vi "LabVIEW2018_RS232_loopback_test.vi"() -> ()   [LabVIEW 2018]
uses:
  <vilib>/Instr/_visa.llb/VISA Configure Serial Port (Instr).vi
panel:
  in  "Delay Time (s)":dbl=0.5 format="%#_13g"
  in  "Send":bool
  in  "Flow control":u16(ring) items=["None", "XON/XOFF", "RTS/CTS", "XON/XOFF & RTS/CTS", "DTR/DSR", "XON/XOFF & DTR/DSR"]
  in  "Stop bits":u16(ring)=10 items=["1.0"=10, "1.5"=15, "2.0"=20]
  in  "Parity":enum16{"None", "Odd", "Even", "Mark", "Space"}(ring)
  in  "Data bits":u16=8
  in  "Baud rate":u32=9600
  in  "Sent Message":string="meas1?"
  in  "VISA resource name":refnum<visa-resource-name>="COM3"
  out "Read Response":string
  in  "stop":bool
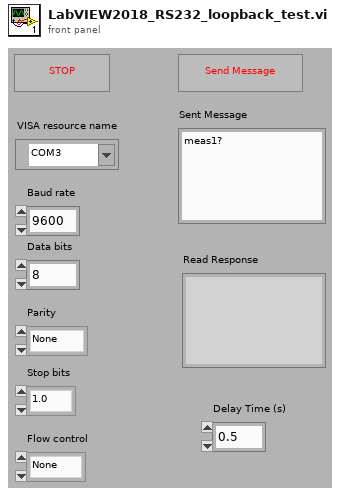
[diagram p1: front panel]
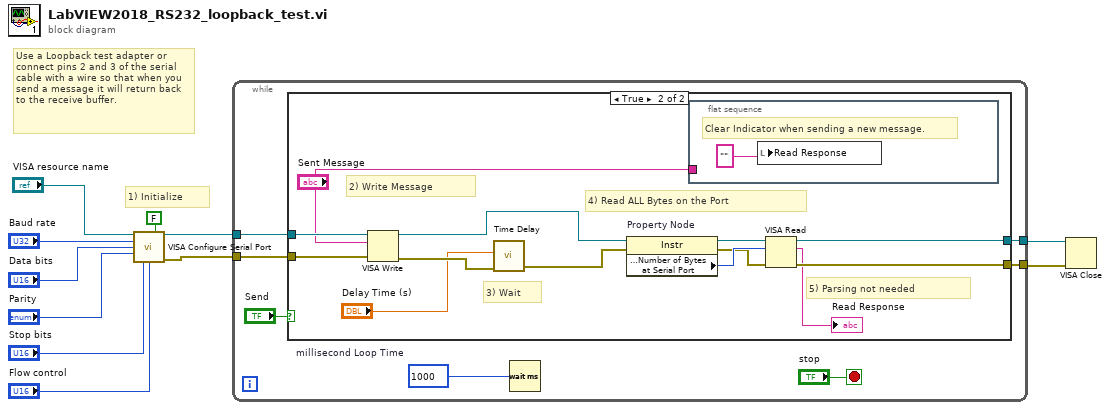
[diagram p0: block diagram]
diagram:
  # "Use a Loopback test adapter or connect pins 2 and 3 of the serial cable with a wire so that when you send a message it will return back to the receive buffer."
  # "1) Initialize"
  n1 = call-poly "VISA Configure Serial Port"("VISA resource name"="VISA resource name", "Enable Termination\nChar (T)"=FALSE ("Enable Termination\nChar (T)"), "baud rate (9600)"="Baud rate", "data bits (8)"="Data bits", "parity (0:none)"="Parity", "stop bits (10: 1 bit)"="Stop bits", "flow control (0:none)"="Flow control") -> ("VISA resource name out"=w5:refnum<visa-resource-name>, "error out"=w4:errorcluster)  [unwired: 1 in, 6 out]
  n2 = while {
    tunnel: w5 -> [w18]
    tunnel: w4 -> [w17]
    tunnel: [w15] -> w3
    tunnel: [w14] -> w2
    stop <- "stop" stop-if-true
    w12 = u32 1000  # millisecond Loop Time
    n3 = case shown="True" "Send" {
      tunnel: w18 -> [w20 w33]
      tunnel: w17 -> [w19 w32]
      tunnel: [w20 w31] -> w15
      tunnel: [w19 w30] -> w14
      frame False {
      }
      frame True {
        # "5) Parsing not needed"
        # "3) Wait"
        # "2) Write Message"
        # "4) Read ALL Bytes on the Port"
        n4 = VISA Write(VISA resource name=w33, write buffer="Sent Message", error in (no error)=w32) -> (VISA resource name out=w24:refnum<visa-resource-name>, error out=w26:errorcluster)  [unwired: 1 out]
        n5 = call "Time Delay"("error in (no error)"=w26, "Delay Time (s)"="Delay Time (s)") -> ("error out"=w25:errorcluster)  [unwired: 9 out]
        n6 = property on="Property Node" class="Instr"(reference=w24, error in=w25) -> (reference out=w28:refnum<visa-resource-name>, error out=w27:errorcluster, "Serial Settings:Number of Bytes at Serial Port"=w29:u32)
        n7 = flat-sequence {
          tunnel: "Sent Message" -> [_]
          frame #0 {
            # "Clear Indicator when sending a new message."
            n8 = local write "Read Response"("" ("Read Response")) -> ()
          }
        }
        n9 = VISA Read(VISA resource name=w28, byte count=w29, error in (no error)=w27) -> (VISA resource name out=w31:refnum<visa-resource-name>, read buffer=→"Read Response":string, error out=w30:errorcluster)  [unwired: 1 out]
      }
    }
    n10 = Wait (ms)(milliseconds to wait=w12) -> ()  [unwired: 1 out]
  }
  n11 = VISA Close(VISA resource name=w3, error in (no error)=w2) -> ()  [unwired: 1 out]
